vi "7.2.vi"() -> ()   [LabVIEW 2017]
panel:
  out "波形图":cluster{dbl[]}[](graph)
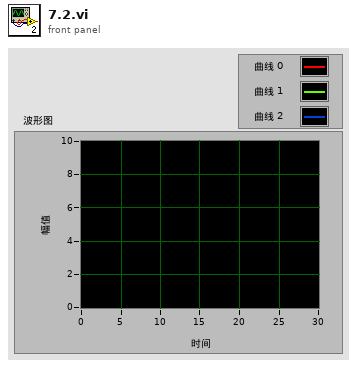
[diagram p1: front panel]
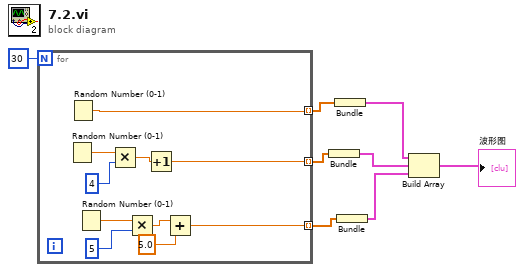
[diagram p0: block diagram]
diagram:
  n1 = for {
    N: 30 -> [_]
    tunnel: [w18] -> w8 mode=indexing
    tunnel: [w10] -> w6 mode=indexing
    tunnel: [w9] -> w7 mode=indexing
    n2 = Random Number (0-1)() -> (number: 0 to 1=w17:dbl)
    n3 = Random Number (0-1)() -> (number: 0 to 1=w18:dbl)
    n4 = Random Number (0-1)() -> (number: 0 to 1=w14:dbl)
    n5 = Multiply(x=w17, y=4) -> (x*y=w15:dbl)
    n6 = Multiply(x=w14, y=5) -> (x*y=w12:dbl)
    n7 = Increment(x=w15) -> (x+1=w9:dbl)
    n8 = Add(x=w12, y=5.0) -> (x+y=w10:dbl)
  }
  n9 = Bundle(w7) -> (w4:cluster{dbl[]})  [unwired: 1 in]
  n10 = Bundle(w8) -> (w5:cluster{dbl[]})  [unwired: 1 in]
  n11 = Bundle(w6) -> (w3:cluster{dbl[]})  [unwired: 1 in]
  n12 = Build Array(w5, w4, w3) -> (→"波形图":cluster{dbl[]}[])
